vi "send_image_processor_update.vi"(8 "error in (no error)":errorcluster, 10 "image processor update":refnum<class "GenericImageProcessor.lvclass">, 11 "DL090216Display in":refnum<class "DisplayDL090216.lvclass">) -> (0 "error out":errorcluster, 3 "DL090216Display out":refnum<class "DisplayDL090216.lvclass">)   [LabVIEW 2010, in "DisplayDL090216.lvclass"]
uses:
  DisplayDL090216.lvclass
  ImageProcessor/GenericImageProcessor/GenericImageProcessor/GenericImageProcessor.lvclass
  action_enum.ctl
  common/classes/ErrorController/ErrorController/class_data.vi
  common/classes/ErrorController/ErrorController/ErrorController.lvclass
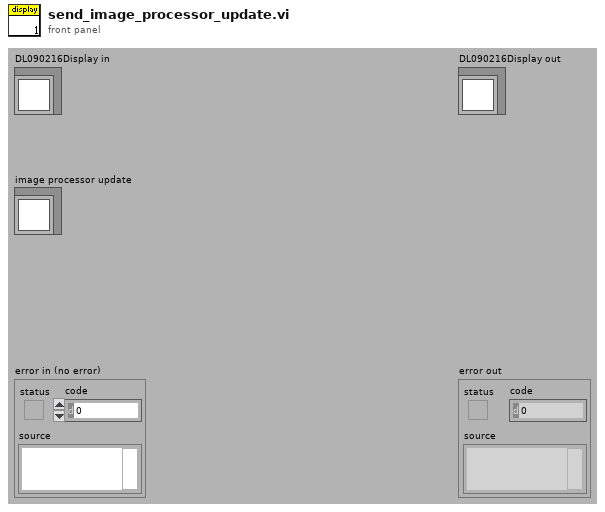
[diagram p1: front panel]
types:
  T1 = typedef "DisplayDL090216.lvclass/action_enum.ctl" = enum16{"NULL", "initialise", "terminate", "fetch", "process", "display", "register as observer"}
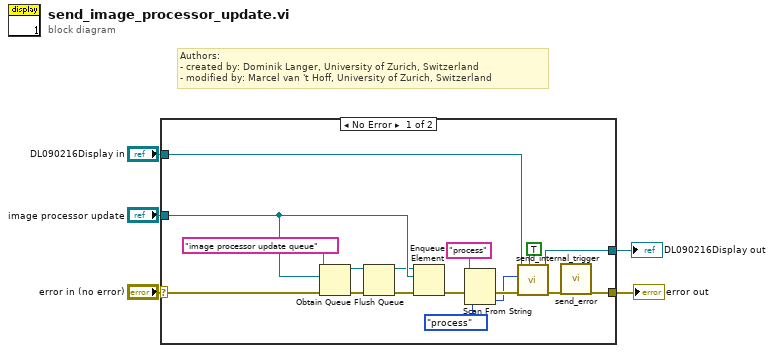
[diagram p0: block diagram]
diagram:
  # "Authors: \n- created by: Dominik Langer, University of Zurich, Switzerland\n- modified by: Marcel van 't Hoff, University of Zurich, Switzerland"
  n1 = case shown="No Error" "error in (no error)" {
    selector: "error in (no error)" -> [w22 w24]
    tunnel: [w11 w24] -> w4
    tunnel: [w18 w23] -> w2
    tunnel: "DL090216Display in" -> [w19 w23]
    tunnel: "image processor update" -> [w20 _]
    frame No Error {
      n2 = Obtain Queue(name (unnamed)="image processor update queue", element data type=w20, error in (no error)=w22) -> (queue out=w14:refnum<queue>, error out=w16:errorcluster)  [unwired: 2 in, 1 out]
      n3 = Flush Queue(queue=w14, error in (no error)=w16) -> (queue out=w13:refnum<queue>, error out=w15:errorcluster)  [unwired: 1 out]
      n4 = Enqueue Element(queue=w13, element=w20, error in (no error)=w15) -> (error out=w9:errorcluster)  [unwired: 3 out]
      n5 = Scan From String(input string="process", error in=w9, default 1=action_enum."process" ("trigger")) -> (error out=w8:errorcluster, output 1=w7:T1)  [unwired: 2 in, 2 out]
      n6 = call-dynamic "send_internal_trigger.vi"("unique insertion?"=TRUE, "error in (no error)"=w8, "trigger"=w7, "DL090216Display in"=w19) -> ("error out"=w12:errorcluster, "DL090216Display out"=w18:refnum<class "DisplayDL090216.lvclass">)  [unwired: 6 out]
      n7 = call "send_error.vi"("error in (no error)"=w12) -> ("error out"=w11:errorcluster)  [unwired: 10 in]
    }
    frame Error {
    }
  }
  "error out" <- w4
  "DL090216Display out" <- w2
